vi "TESTE CURVA GRUPO-4.vi"() -> ()   [LabVIEW 2014]
uses:
  <vilib>/Platform/TimedLoop/XDataNode/timing_clust.ctl
  <vilib>/Platform/TimedLoop/XDataNode/nitl_modes.ctl
  <vilib>/Platform/TimedLoop/XDataNode/wakeup.ctl
  <vilib>/Platform/TimedLoop/XDataNode/XDataNode.xnode
  <userlib>/Newport ESP301/Newport ESP301.lvlib
  <vilib>/Platform/TimedLoop/XDataNode/XDNodeRunTimeDep.lvlib
panel:
  out "x*y":dbl
  out "sin(x)":dbl
  in  "L":dbl=10.0 format="%.1f"
  in  "In.Curva":dbl=2.0
  in  "Raio":dbl=50.0
  out "Yin":dbl format="%.6g"
  out "Xin":dbl format="%.6g"
  out "d (um)":dbl
  in  "d (um)":dbl=100.0
  in  "Stop Button":bool
  out "error out":errorcluster
  out "X (mm)":dbl format="%.2g"
  out "Y (um)":dbl format="%.1f"
  out "XY Graph":cluster{dbl[], dbl[]}(graph)={[0.0, 0.0, 0.0, 0.0, 0.0, 0.0, 0.0, 0.0, 0.0, 0.0, 0.0, 0.0, 0.0, 0.0, 0.0, 0.0, 0.0, 0.0, 0.0, 0.0, 0.0, 0.0, 0.0, 0.0, 0.0, 0.0, 0.0, 0.0, 0.0, 0.0, 0.0, 0.0, 0.0, 0.0, 0.0, 0.0, 0.0, 0.0, 0.0, 0.0, 0.0, 0.0, 0.0, 0.0, 0.0, 0.0, 0.0, 0.0, 0.0, 0.0, 0.0, 0.0, 0.0, 0.0, 0.0, 0.0, 0.0, 0.0, 0.0, 0.0, 0.0, 0.0, 0.0, 0.0, 0.0, 0.0, 0.0, 0.0, 0.0, 0.0, 0.0, 0.0, 0.0, 0.0, 0.0, 0.0], [4600.0, 4600.0, 4600.0, 4600.0, 4600.0, 4600.0, 4600.0, 4600.0, 4600.0, 4600.0, 4600.0, 4600.0, 4600.0, 4600.0, 4600.0, 4600.0, 4600.0, 4600.0, 4600.0, 4600.0, 4600.0, 4600.0, 4600.0, 4600.0, 4600.0, 4600.0, 4600.0, 4690.0, 4802.5, 4800.5, 4799.5, 4799.5, 4799.5, 4800.0, 4800.0, 4800.0, 4800.0, 4800.0, 4800.0, 4800.0, 4800.0, 4800.0, 4800.0, 4800.0, 4995.5, 5001.5, 5000.5, 5000.0, 5000.0, 4999.5, 4999.5, 5000.0, 5000.0, 5000.0, 5000.0, 5000.0, 5000.0, 5000.0, 5000.0, 5000.0, 5000.0, 5000.0, 5000.0, 5000.0, 5000.0, 5000.0, 5000.0, 5000.0, 5000.0, 5000.0, 5000.0, 5000.0, 5000.0, 5000.0, 5000.0, 5000.0]}
  in  "Refresh Button":bool
  in  "Velocity":dbl=3.0
  # "Inicio curva"
  # "Tamanho da amostra (mm)"
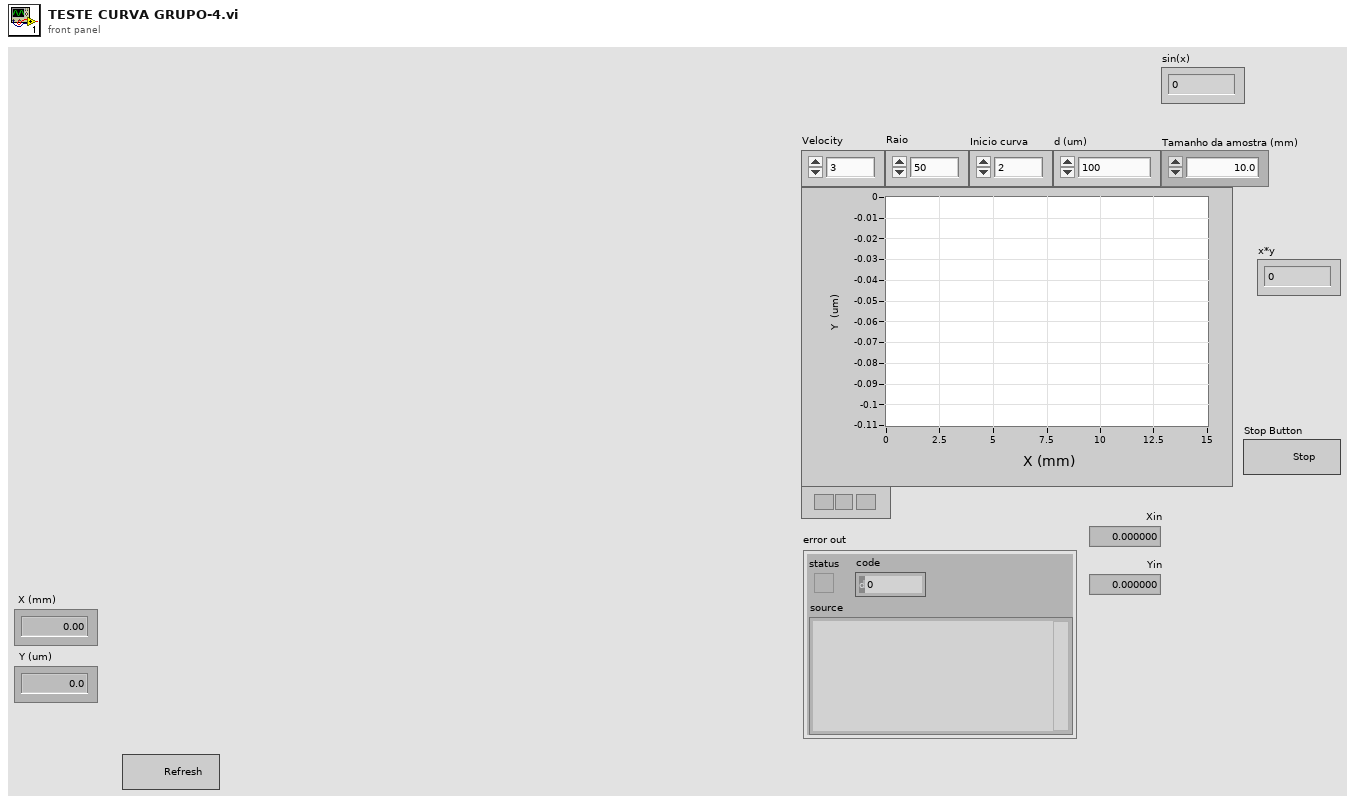
[diagram p1: front panel]
types:
  T1 = typedef "XDNodeRunTimeDep.lvlib/timing_clust.ctl" = cluster{"Expected End [f-1]":u64, "Actual End [f-1]":u64, "Finished Late? [f-1]":bool, "Expected End [i-1]":u64, "Actual End [i-1]":u64, "Finished Late? [i-1]":bool, "Expected Start [i]":u64, "Actual Start [i]":u64, "Expected Start [f]":u64, "Actual Start [f]":u64, "Source Name":string, "Structure Name":string, "Period":i64, "Deadline":i64, "Offset":i64, "Start":i64, "Priority":i32, "Timeout":i32, "Mode":T2, "Wakeup Reason":T3, "Error":errorcluster, "Source Type":string, "Secondary Source Type":string, "Global End Time":u64, "Global Start Time":u64, "Frame Duration":u64, "Iteration Duration":u64, "Assigned CPU":i32, "I/O Scan Engine Mode":u32}
  T2 = typedef "XDNodeRunTimeDep.lvlib/nitl_modes.ctl" = enum32{"No Change", "Process missed periods, maintain original phase", "Discard missed periods, maintain original phase", "Process missed periods, ignore original phase", "Discard missed periods, ignore original phase"}
  T3 = typedef "XDNodeRunTimeDep.lvlib/wakeup.ctl" = enum32{"Normal", "Aborted", "Asynchronous wakeup", "Timing source error", "Timed loop error", "Timeout"}
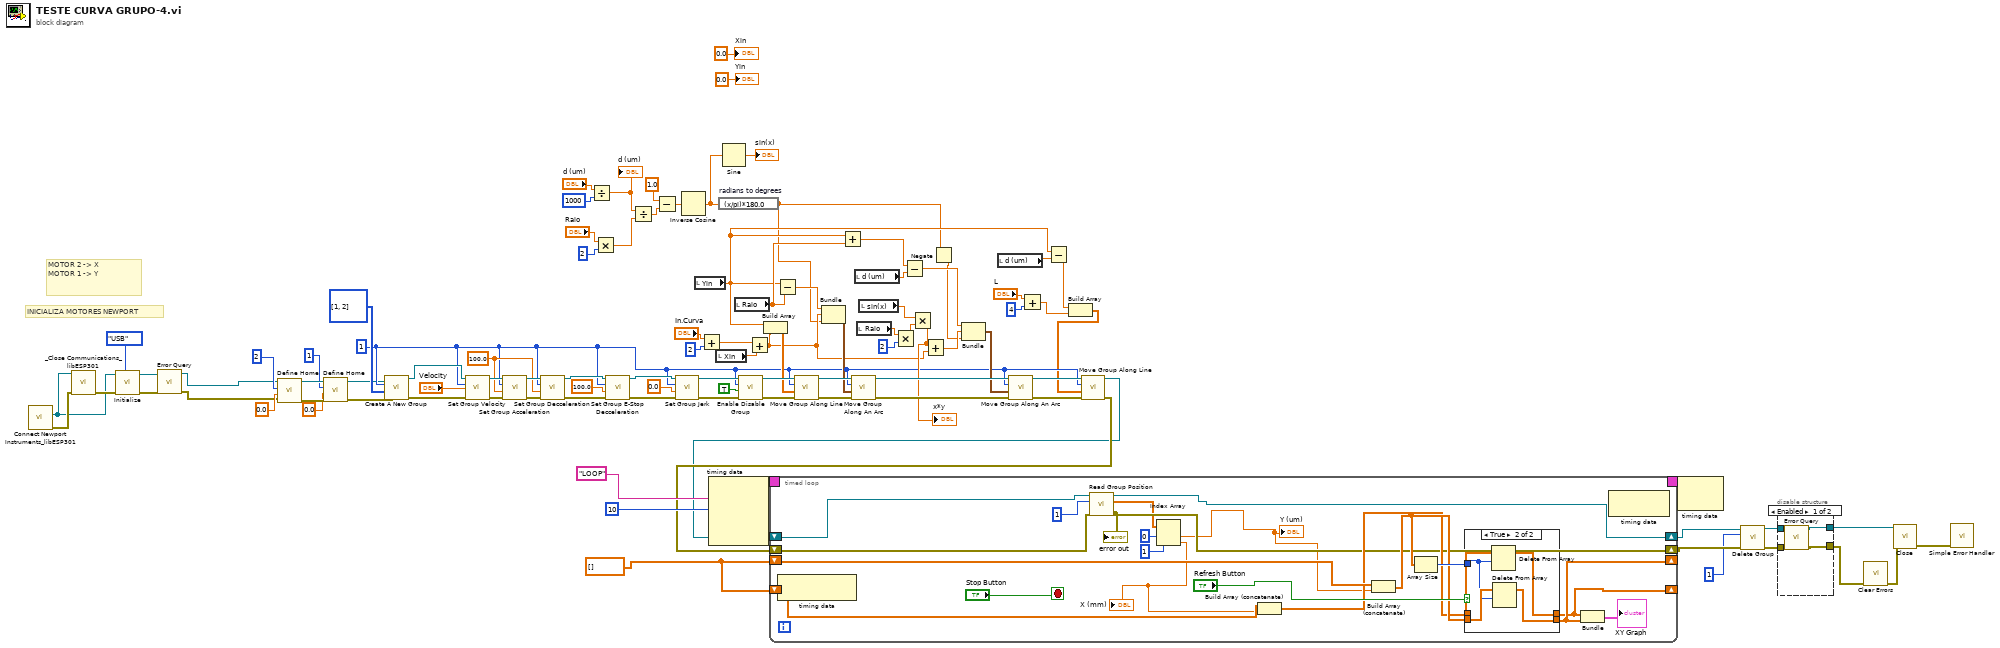
[diagram p0: block diagram]
diagram:
  w69 = dbl[] []
  w18 = 1 ("Group #")
  w88 = 100.0 ("Acceleration (0 units/s²)")
  # "MOTOR 2 -> X\nMOTOR 1 -> Y"
  # "INICIALIZA MOTORES NEWPORT"
  n1 = call <userlib>:"Connect Newport Instruments_libESP301.vi"() -> ("error (duplicate)"=w98:errorcluster, "VISA resource name (duplicate)"=w97:refnum<visa-resource-name>)  [unwired: 7 in, 3 out]
  n2 = call <userlib>:"_Close Communications_libESP301.vi"("Instrument Channel"=w97, "error in (no error)"=w98) -> ("error out"=w100:errorcluster)  [unwired: 13 in]
  n3 = call <userlib>:"Initialize.vi"("VISA resource name"=w97, "error in (no error)"=w100, "Serial Link (RS232)"=enum16{"RS232", "USB"}."USB") -> ("VISA resource name out"=w78:refnum<visa-resource-name>, "error out"=w77:errorcluster)  [unwired: 6 in]
  n4 = call <userlib>:"Error Query.vi"("error in (no error)"=w77, "VISA resource name"=w78) -> ("error out"=w3:errorcluster, "VISA resource name out"=w4:refnum<visa-resource-name>)  [unwired: 2 in, 2 out]
  n5 = call <userlib>:"Define Home.vi"("error in (no error)"=w3, "Home Position (0 units)"=0.0, "Axis (1)"=2 ("y"), "VISA resource name"=w4) -> ("error out"=w9:errorcluster, "VISA resource name out"=w10:refnum<visa-resource-name>)  [unwired: 2 in]
  n6 = call <userlib>:"Define Home.vi"("error in (no error)"=w9, "Home Position (0 units)"=0.0, "Axis (1)"=1, "VISA resource name"=w10) -> ("error out"=w1:errorcluster, "VISA resource name out"=w2:refnum<visa-resource-name>)  [unwired: 2 in]
  n7 = call <userlib>:"Create A New Group.vi"("error in (no error)"=w1, "Axis Number"=i32[] [1, 2], "Group Number (1)"=w18, "VISA resource name"=w2) -> ("error out"=w94:errorcluster, "VISA resource name out"=w95:refnum<visa-resource-name>)  [unwired: 2 in]
  n8 = call <userlib>:"Set Group Velocity.vi"("error in (no error)"=w94, "Velocity (units/s)"="Velocity", "Group Number (1)"=w18, "VISA resource name"=w95) -> ("error out"=w89:errorcluster, "VISA resource name out"=w92:refnum<visa-resource-name>)  [unwired: 2 in]
  n9 = call <userlib>:"Set Group Acceleration.vi"("error in (no error)"=w89, "Acceleration (0 units/s²)"=w88, "Group Number (1)"=w18, "VISA resource name"=w92) -> ("error out"=w90:errorcluster, "VISA resource name out"=w91:refnum<visa-resource-name>)  [unwired: 2 in]
  n10 = call <userlib>:"Set Group Decceleration.vi"("error in (no error)"=w90, "Decceleration (0 units/s²)"=w88, "Group Number (1)"=w18, "VISA resource name"=w91) -> ("error out"=w84:errorcluster, "VISA resource name out"=w87:refnum<visa-resource-name>)  [unwired: 2 in]
  n11 = Divide(x="d (um)", y=1000) -> (x/y=w49:dbl)
  "d (um)" <- w49
  n12 = Multiply(x="Raio", y=2) -> (x*y=w58:dbl)
  n13 = call <userlib>:"Set Group E-Stop Decceleration.vi"("error in (no error)"=w84, "E-Stop Decceleration (0 units/s²)"=100.0, "Group Number (1)"=w18, "VISA resource name"=w87) -> ("error out"=w83:errorcluster, "VISA resource name out"=w86:refnum<visa-resource-name>)  [unwired: 2 in]
  n14 = Divide(x=w49, y=w58) -> (x/y=w53:dbl)
  n15 = Subtract(x=1.0, y=w53) -> (x-y=w51:dbl)
  n16 = call <userlib>:"Set Group Jerk.vi"("error in (no error)"=w83, "Vector Jerk (0 units/s^3)"=0.0, "Group Number (1)"=w18, "VISA resource name"=w86) -> ("error out"=w82:errorcluster, "VISA resource name out"=w85:refnum<visa-resource-name>)  [unwired: 2 in]
  n17 = Inverse Cosine(1:w51) -> (0:w36:dbl)
  n18 = local read "Yin"() -> (w15:dbl)
  n19 = Add(x="In.Curva", y=2) -> (x+y=w34:dbl)
  n20 = node-c288("LOOP" ("Structure Name"), i64 10 ("Period")) -> (w73:T1)  [unwired: 2 in]
  n21 = local read "Xin"() -> (w38:dbl)
  n22 = expression code="(x/pi)*180.0" "radians to degrees"(w36) -> (w12:dbl)
  n23 = Sine(x=w36) -> (sin(x)=→"sin(x)":dbl)
  n24 = local read "Raio"() -> (w26:dbl)
  n25 = call <userlib>:"Enable Disable Group.vi"("error in (no error)"=w82, "Action (OFF)"=TRUE, "Group Number (1)"=w18, "VISA resource name"=w85) -> ("error out"=w47:errorcluster, "VISA resource name out"=w48:refnum<visa-resource-name>)  [unwired: 2 in]
  n26 = Add(x=w34, y=w38) -> (x+y=w28:dbl)
  n27 = Build Array(w15, w28) -> (w44:dbl[])
  n28 = Subtract(x=w15, y=w26) -> (x-y=w37:dbl)
  n29 = call <userlib>:"Move Group Along Line.vi"("error in (no error)"=w47, "Position (0 units)"=w44, "Group Number (1)"=w18, "VISA resource name"=w48) -> ("error out"=w42:errorcluster, "VISA resource name out"=w43:refnum<visa-resource-name>)  [unwired: 2 in]
  n30 = Bundle(w37, w28, w12) -> (w41:cluster{dbl, dbl, dbl})  [unwired: 1 in]
  n31 = Add(x=w15, y=w26) -> (x+y=w25:dbl)
  n32 = call <userlib>:"Move Group Along An Arc.vi"("error in (no error)"=w42, "Arc  Parameters"=w41, "Group Number (1)"=w18, "VISA resource name"=w43) -> ("error out"=w75:errorcluster, "VISA resource name out"=w76:refnum<visa-resource-name>)  [unwired: 2 in]
  n33 = local read "d (um)"() -> (w24:dbl)
  n34 = local read "Raio"() -> (w32:dbl)
  n35 = local read "sin(x)"() -> (w31:dbl)
  n36 = Multiply(x=w32, y=2) -> (x*y=w30:dbl)
  n37 = Subtract(x=w25, y=w24) -> (x-y=w23:dbl)
  n38 = Multiply(x=w31, y=w30) -> (x*y=w29:dbl)
  "x*y" <- w29
  n39 = Add(x=w29, y=w28) -> (x+y=w27:dbl)
  n40 = Negate(x=w12) -> (-x=w11:dbl)
  n41 = Bundle(w23, w27, w11) -> (w74:cluster{dbl, dbl, dbl})  [unwired: 1 in]
  n42 = local read "d (um)"() -> (w16:dbl)
  n43 = call <userlib>:"Move Group Along An Arc.vi"("error in (no error)"=w75, "Arc  Parameters"=w74, "Group Number (1)"=w18, "VISA resource name"=w76) -> ("error out"=w21:errorcluster, "VISA resource name out"=w22:refnum<visa-resource-name>)  [unwired: 2 in]
  n44 = Add(x="L", y=4) -> (x+y=w17:dbl)
  n45 = Subtract(x=w15, y=w16) -> (x-y=w14:dbl)
  n46 = Build Array(w14, w17) -> (w13:dbl[])
  n47 = call <userlib>:"Move Group Along Line.vi"("error in (no error)"=w21, "Position (0 units)"=w13, "Group Number (1)"=w18, "VISA resource name"=w22) -> ("error out"=w20:errorcluster, "VISA resource name out"=w19:refnum<visa-resource-name>)  [unwired: 2 in]
  n48 = timed-loop {
    timing: w73 -> [_]
    timing-out: [_] -> w72
    shift-right: [w108] -> w64
    shift-left: w19 -> [w110]
    shift-right: [w107] -> w63
    shift-left: w20 -> [w109]
    shift-right: [w113] -> _
    shift-left: w69 -> [w117]
    shift-right: [w112] -> _
    shift-left: w69 -> [w115]
    stop <- "Stop Button" stop-if-true
    n49 = node-c288() -> ()  [unwired: 1 in, 1 out]
    n50 = call <userlib>:"Read Group Position.vi"("error in (no error)"=w109, "Group Number (1)"=1, "VISA resource name"=w110) -> ("error out"=w107:errorcluster, "Position (units)"=w104:dbl[], "VISA resource name out"=w108:refnum<visa-resource-name>)  [unwired: 2 in]
    "error out" <- w107
    n51 = Index Array(array=w104, index #1=0 ("index"), index #2=1 ("index")) -> (element #1=w103:dbl, element #2=w102:dbl)
    "X (mm)" <- w102
    "Y (um)" <- w103
    n52 = Build Array (concatenate)(w115, w102) -> (w114:dbl[])
    n53 = Build Array (concatenate)(w117, w103) -> (w116:dbl[])
    n54 = Array Size(array=w116) -> (size(s)=w118:i32)
    n55 = case shown="True" "Refresh Button" {
      tunnel: [w122 w124] -> w112
      tunnel: w114 -> [w122 w127]
      tunnel: [w121 w123] -> w113
      tunnel: w116 -> [w121 w126]
      tunnel: w118 -> [_ w125]
      frame False {
      }
      frame True {
        n56 = Delete From Array(array=w127, length=w125) -> (array with subset deleted=w124:dbl[])  [unwired: 1 in, 1 out]
        n57 = Delete From Array(array=w126, length=w125) -> (array with subset deleted=w123:dbl[])  [unwired: 1 in, 1 out]
      }
    }
    n58 = Bundle(w112, w113) -> (→"XY Graph":cluster{dbl[], dbl[]})  [unwired: 1 in]
    n59 = node-c288() -> ()  [unwired: 1 in, 1 out]
  }
  n60 = node-c288(w72) -> ()  [unwired: 1 out]
  n61 = call <userlib>:"Delete Group.vi"("error in (no error)"=w63, "Group Number (1)"=1, "VISA resource name"=w64) -> ("error out"=w67:errorcluster, "VISA resource name out"=w68:refnum<visa-resource-name>)  [unwired: 3 in]
  n62 = disable-structure shown="Enabled" {
    disable-tunnel: w68 -> [w133 w135]
    disable-tunnel: w67 -> [w132 w134]
    disable-tunnel: [w131 w135] -> w66
    disable-tunnel: [w130 w134] -> w61
    frame Enabled {
      n63 = call <userlib>:"Error Query.vi"("error in (no error)"=w132, "VISA resource name"=w133) -> ("error out"=w130:errorcluster, "VISA resource name out"=w131:refnum<visa-resource-name>)  [unwired: 2 in, 2 out]
    }
    frame Disabled {
    }
  }
  n64 = call <vilib>:"Clear Errors.vi"("error in (no error)"=w61) -> ("error out"=w60:errorcluster)  [unwired: 5 in, 1 out]
  n65 = call <userlib>:"Close.vi"("error in (no error)"=w60, "VISA resource name"=w66) -> ("error out"=w65:errorcluster)  [unwired: 9 in]
  n66 = call <vilib>:"Simple Error Handler.vi"("error in (no error)"=w65) -> ()  [unwired: 4 in, 5 out]
  "Xin" <- 0.0 ("Xin")
  "Yin" <- 0.0 ("Yin")
